vi "ppms_TH_control_v2.vi"(0 "ppms control ?":bool=TRUE, 5 "wait T status":bool, 7 "radio":enum32{"or", "and"}(radio)=enum."and", 9 "wait H status":bool, 11 "error in (no error)":errorcluster caption="entrée d'erreur (pas d'erreur)") -> (2 "Temperature (K)":dbl format="%.3f", 3 "T /K":dynamicdata(graph), 4 "go to next state":bool=TRUE, 6 "Temperature Status":string, 8 "Magnet Status":string, 13 "Field (Oe)":dbl format="%.3f", 14 "H":dynamicdata(graph), 15 "error out":errorcluster caption="sortie d'erreur")   [LabVIEW 2018]
doc: "Utilisez ce modèle pour construire un VI à utiliser en tant que sous-VI."
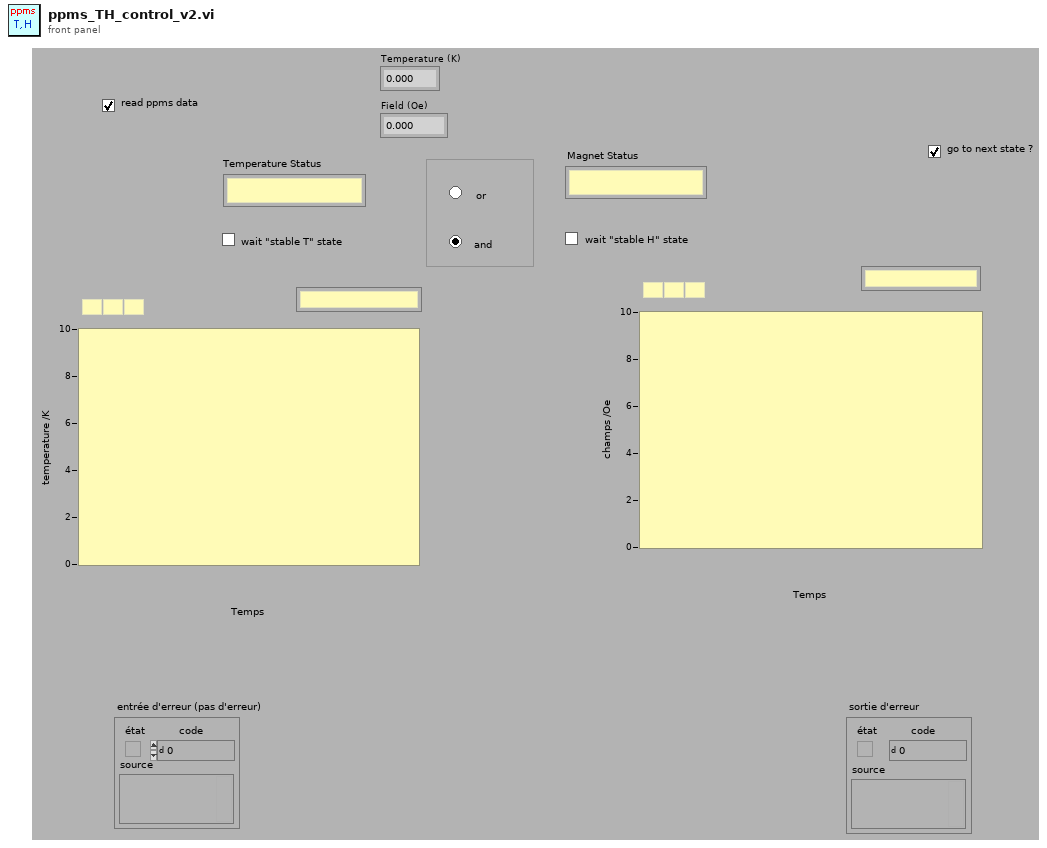
[diagram p1: front panel]
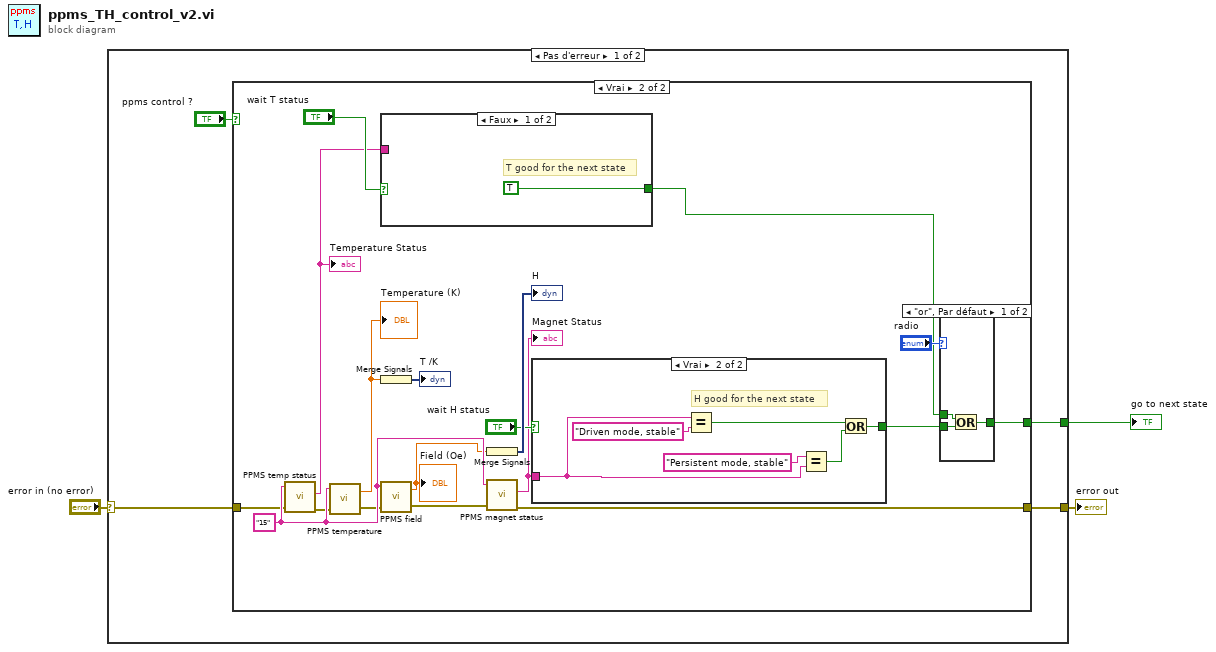
[diagram p0: block diagram]
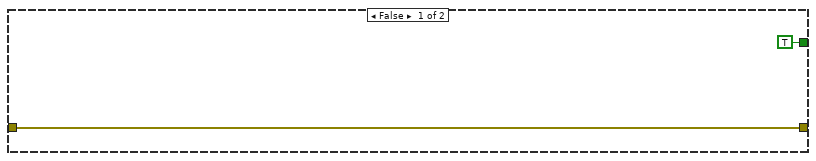
[diagram p2: hidden frame]
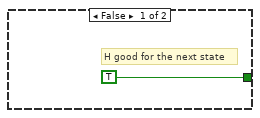
[diagram p3: hidden frame]
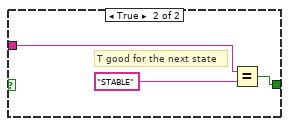
[diagram p4: hidden frame]
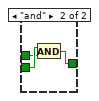
[diagram p5: hidden frame]
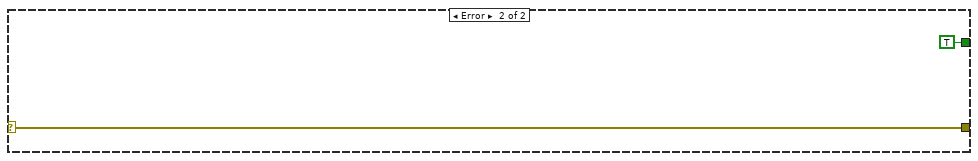
[diagram p6: hidden frame]
diagram:
  n1 = case shown="Pas d'erreur" "error in (no error)" {
    selector: "error in (no error)" -> [w5 w46]
    tunnel: [w4 w46] -> w2
    tunnel: [w6 TRUE ("wait T status")] -> w1
    frame No Error {
      n2 = case shown="Vrai" "ppms control ?" {
        tunnel: [TRUE ("wait T status") w16] -> w6
        tunnel: w5 -> [w8 w18]
        tunnel: [w8 w17] -> w4
        frame False {
        }
        frame True {
          w27 = "15" ("PPMS GPIB address")
          n3 = call "PPMS temp status.vi"("GPIB address"=w27, "error in (no error)"=w18) -> ("Temperature Status"=w14:string, "error out"=w26:errorcluster)  [unwired: 1 in, 2 out]
          "Temperature Status" <- w14
          n4 = call "PPMS temperature.vi"("error in (no error)"=w26, "GPIB address"=w27) -> ("error out"=w25:errorcluster, "Temperature (K)"=w23:dbl)  [unwired: 1 in]
          "Temperature (K)" <- w23
          n5 = case shown="Faux" "wait T status" {
            tunnel: w14 -> [_ w37]
            tunnel: [TRUE w36] -> w13
            frame False {
              # "T good for the next state"
            }
            frame True {
              # "T good for the next state"
              n6 = Equal?(x=w37, y="STABLE") -> (x = y?=w36:bool)
            }
          }
          n7 = Merge Signals(w23) -> (→"T /K":dynamicdata)
          n8 = call "PPMS field.vi"("error in (no error)"=w25, "GPIB address"=w27) -> ("error out"=w24:errorcluster, "Field (Oe)"=w22:dbl)  [unwired: 1 in]
          "Field (Oe)" <- w22
          n9 = Merge Signals(w22) -> (→"H":dynamicdata)
          n10 = call "PPMS magnet status.vi"("GPIB address"=w27, "error in (no error)"=w24) -> ("Magnet Status"=w11:string, "error out"=w17:errorcluster)  [unwired: 1 in, 2 out]
          "Magnet Status" <- w11
          n11 = case shown="Vrai" "wait H status" {
            tunnel: [TRUE w30] -> w10
            tunnel: w11 -> [_ w29]
            frame False {
              # "H good for the next state"
            }
            frame True {
              # "H good for the next state"
              n12 = Equal?(x=w29, y="Driven mode, stable") -> (x = y?=w33:bool)
              n13 = Equal?(x="Persistent mode, stable", y=w29) -> (x = y?=w32:bool)
              n14 = Or(x=w33, y=w32) -> (x .or. y?=w30:bool)
            }
          }
          n15 = case shown="\"or\", Par défaut" "radio" {
            tunnel: [w41 w44] -> w16
            tunnel: w13 -> [w40 w42]
            tunnel: w10 -> [w39 w43]
            frame "or", Default {
              n16 = Or(x=w40, y=w39) -> (x .or. y?=w41:bool)
            }
            frame "and" {
              n17 = And(x=w43, y=w42) -> (x .and. y?=w44:bool)
            }
          }
        }
      }
    }
    frame Error {
    }
  }
  "error out" <- w2
  "go to next state" <- w1
